vi "MT Generate PAM system parameters (map).vi"(0 "samples per symbol (16)":i32=16, 5 "symbol values":i32[](array[numeric]), 11 "error in (no error)":errorcluster) -> (6 "PAM system parameters":T1 {"symbol map" format="%.3f"}, 8 "bits per symbol":i32, 15 "error out":errorcluster)   [LabVIEW 2020, in "niDMT.lvlib"]
doc: "This polymorphic instance calculates parameters for use with either the MT Modulate PAM VI or the MT Demodulate PAM VI. It accepts an array of <B>symbol values</B> that explicitly specifies the positions of the symbol map with symbols that are evenly distributed between &#8211;1 and 1."
uses:
  <vilib>/addons/Modulation/niDMT.lvlib
  <vilib>/addons/Modulation/Digital/Support/Controls/PAM system parameters.ctl
  <vilib>/addons/Modulation/niAMT.lvlib
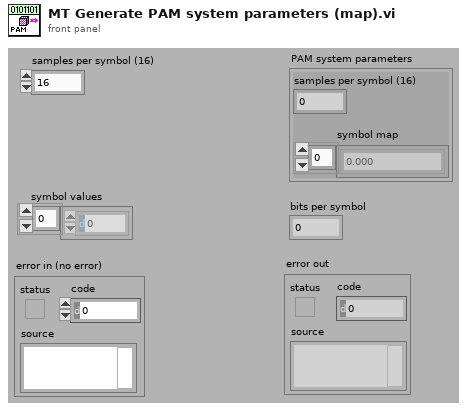
[diagram p1: front panel]
types:
  T1 = cluster{"samples per symbol (16)":i32, "symbol map":cdb[]}
  T2 = typedef "niDMT.lvlib/PAM system parameters.ctl" = cluster{"samples per symbol (16)":i32, "symbol map":cdb[]}
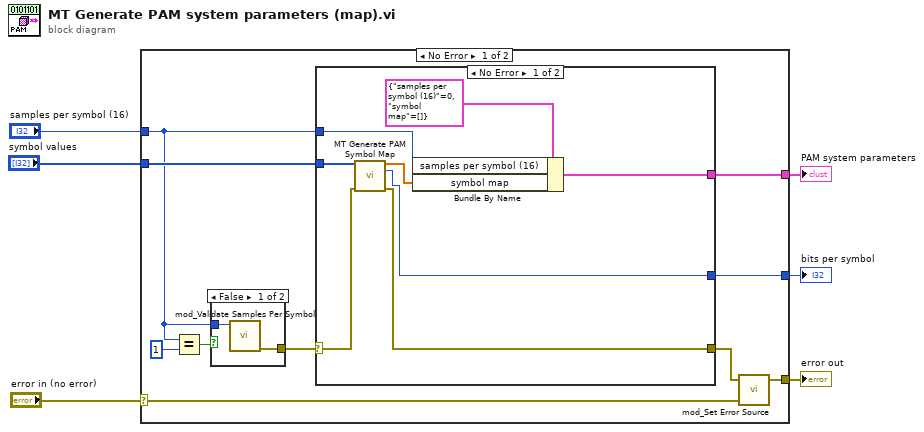
[diagram p0: block diagram]
diagram:
  n1 = case shown="No Error" "error in (no error)" {
    selector: "error in (no error)" -> [w12 w28]
    tunnel: "samples per symbol (16)" -> [w9 _]
    tunnel: "symbol values" -> [w16 _]
    tunnel: [w15 _] -> w4
    tunnel: [w14 _] -> w3
    tunnel: [w11 w28] -> w2
    frame No Error {
      n2 = Equal?(x=w9, y=1) -> (x = y?=w7:bool)
      n3 = case shown="False" w7 {
        tunnel: w9 -> [w18 _]
        tunnel: [w17 _] -> w13
        frame False {
          n4 = call <vilib>:"mod_Validate Samples Per Symbol.vi"("Samples Per Symbol"=w18) -> ("error out"=w17:errorcluster)  [unwired: 10 out]
        }
        frame True {
        }
      }
      n5 = case shown="No Error" w13 {
        selector: w13 -> [w19 w27]
        tunnel: w16 -> [w24 _]
        tunnel: [w23 _] -> w15
        tunnel: [w22 _] -> w14
        tunnel: [w21 w27] -> w10
        tunnel: w9 -> [w20 _]
        frame No Error {
          n6 = call <vilib>:"MT Generate PAM Symbol Map.vi"("symbol values"=w24, "error in (no error)"=w19) -> ("symbol map"=w25:cdb[], "bits per symbol"=w22:i32, "error out"=w21:errorcluster)  [unwired: 11 out]
          n7 = Bundle By Name(cluster=T2 {"samples per symbol (16)"=0, "symbol map"=[]} ("PAM System Parameters"), "samples per symbol (16)"=w20, "symbol map"=w25) -> (w23:T2)
        }
        frame Error {
        }
      }
      n8 = call <vilib>:"mod_Set Error Source.vi"("initial error in (no error)"=w12, "final error in (no error)"=w10) -> ("error out"=w11:errorcluster)  [unwired: 3 out]
    }
    frame Error {
    }
  }
  "PAM system parameters" <- w4
  "bits per symbol" <- w3
  "error out" <- w2
